vi "Create Data Channels.vi"(8 "error in":errorcluster, 11 "Node in":refnum<class "BLS Cycler Template.lvclass">) -> (0 "error out":errorcluster, 3 "Node out":refnum<class "BLS Cycler Template.lvclass">)   [LabVIEW 2023, in "BLS Cycler Template.lvlib" / "BLS Cycler Template.lvclass"]
uses:
  BLS Cycler Template.lvclass
  BLS Cycler Template.lvclass/BLS Cycler Template.ctl
  <vilib>/ADAS Replay HIL/Template Node/Plugin/Template Node/Template Node.lvclass
  bls-capabilities/src/Capabilities/High Level Capabilities/Cycler/Cycler.lvclass
  C:/Program Files/National Instruments/LabVIEW 2023/vi.lib/ADAS Replay HIL/Template Node/Plugin/Template Node/Template Node.lvclass
  C:/Program Files/National Instruments/ADAS Replay HIL/EVO SDK/Linux RT/evoLabVIEWAPI/evoBlockPlugin.lvlibp/evoBlockPlugin/BlockPluginInterface.2020.1/BlockPluginInterface.2020.1.lvclass
  C:/Users/amomin/BLS/bls-cycler-plugin-template/src/Plugin/BLS Cycler Template/BLS Cycler Template.lvclass
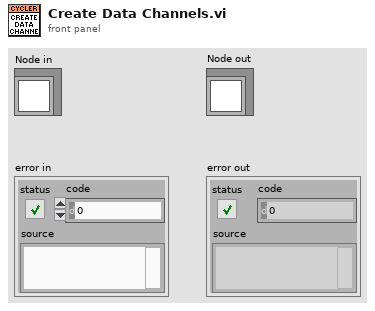
[diagram p1: front panel]
types:
  T1 = typedef "BLS Cycler Template.lvlib/BLS Cycler Template.lvclass/Configuration Params.ctl" = cluster{"Common":T2, "Amount of Channels":u32, "Address":string}
  T2 = typedef "Template Node.lvlib/Template Node.lvclass/Common Configuration Params.ctl" = cluster{"Iteration Interval (s)":dbl, "T0 (ns)":u64, "Priority":i32, "Processor":i32, "Wait in Ready State":bool}
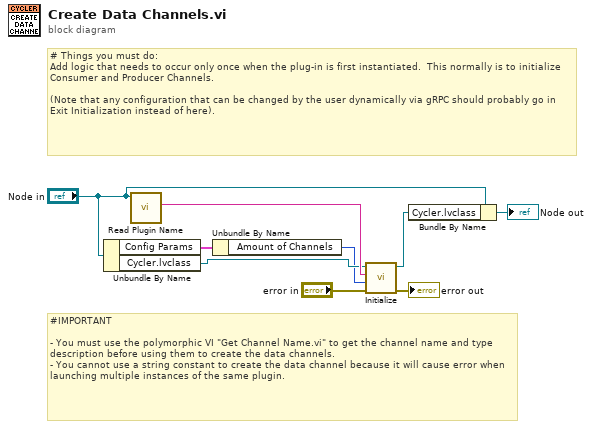
[diagram p0: block diagram]
diagram:
  # "# Things you must do:\nAdd logic that needs to occur only once when the plug-in is first instantiated.  This normally is to initialize Consumer and Producer Channels.   \n\n(Note that any configuration that can be changed by the user dynamically via gRPC should probably go in Exit Initialization instead of here)."
  # "#IMPORTANT\n\n- You must use the polymorphic VI \"Get Channel Name.vi\" to get the channel name and type description before using them to create the data channels.\n- You cannot use a string constant to create the data channel because it will cause error when launching multiple instances of the same plugin."
  n1 = Unbundle By Name("Node in") -> ("Config Params"=w9:T1, "Cycler.lvclass"=w5:refnum<class "Cycler.lvclass">)
  n2 = call <vilib>:"Read Plugin Name.vi"("Template Node in"="Node in") -> ("Plugin Name"=w6:string)  [unwired: 8 in, 2 out]
  n3 = Unbundle By Name(w9) -> ("Amount of Channels"=w2:u32)
  n4 = call-dynamic "Initialize.vi"("error in"="error in", "Number of Channels"=w2, "Instance Name"=w6, "Cycler in"=w5) -> ("error out"=→"error out":errorcluster, "Cycler out"=w8:refnum<class "Cycler.lvclass">)  [unwired: 6 in]
  n5 = Bundle By Name(cluster="Node in", "Cycler.lvclass"=w8) -> (→"Node out":refnum<class "BLS Cycler Template.lvclass">)
